vi "Select Device.vi"(2 "error in (no error)":errorcluster, 3 "Device":i32) -> (0 "error out":errorcluster, 1 "function return":i32)   [LabVIEW 2014, in "ThorZStepper.lvlib"]
doc: "long SelectDevice(const long Device);"
uses:
  ThorZStepper.lvlib
  ThorZStepper.dll
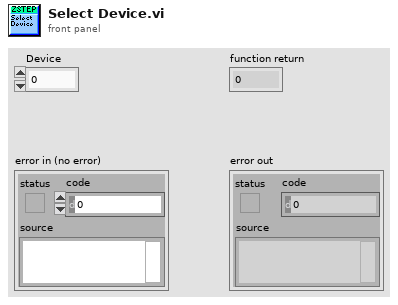
[diagram p1: front panel]
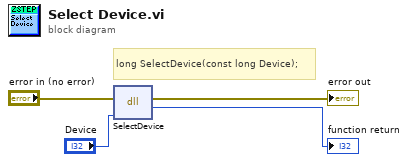
[diagram p0: block diagram]
diagram:
  # "long SelectDevice(const long Device);"
  n1 = dll-call lib="C:/TIS_CalebVS2012/TIS_Development/Hardware/SDKs/MFC1_SDK/LabVIEW/inc/ThorZStepper.*" fn="SelectDevice"(error in="error in (no error)", "Device"="Device") -> (error out=→"error out":errorcluster, "return type"=→"function return":i32)  [unwired: 3 in, 1 out]
